vi "LJstreamM parse formula.vi"(7 "Num Args":u32, 8 "error in (no error)":errorcluster, 11 "Input Formula":string) -> (0 "error out":errorcluster, 2 "Output Formula Arguments":string[](array[string]), 3 "Output Formula":string)   [LabVIEW 2022 SP3]
doc: "Similar to the Formula Node function, but with variables that can be entered on the front panel."
panel:
  out "before substring 2":string
  out "before substring":string
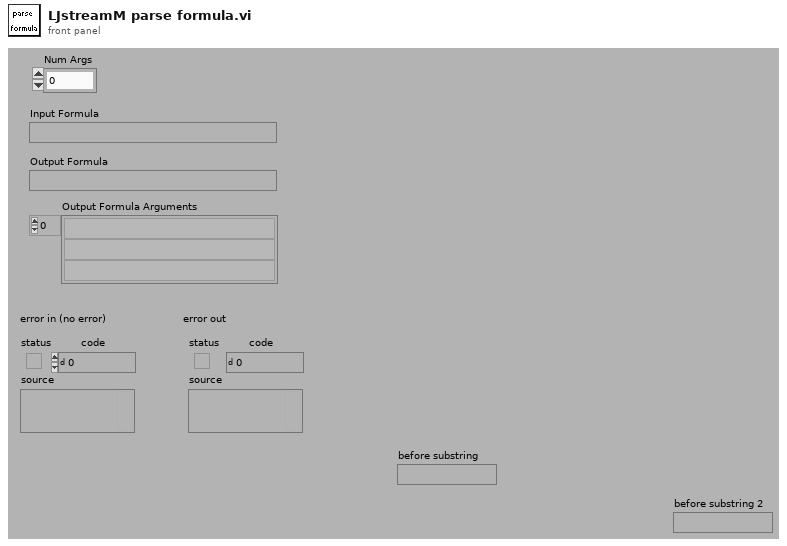
[diagram p1: front panel]
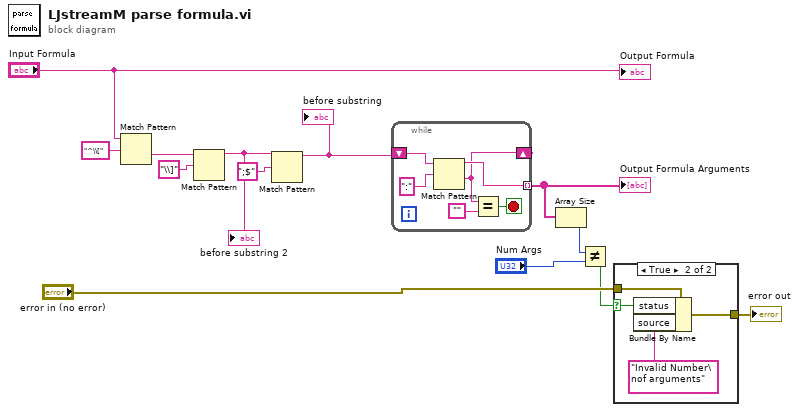
[diagram p0: block diagram]
diagram:
  n1 = Match Pattern(string="Input Formula", regular expression="^\\[") -> (after substring=w11:string)  [unwired: 1 in, 3 out]
  n2 = Match Pattern(string=w11, regular expression="\\]") -> (before substring=w2:string)  [unwired: 1 in, 3 out]
  "before substring 2" <- w2
  n3 = Match Pattern(string=w2, regular expression=";$") -> (before substring=w1:string)  [unwired: 1 in, 3 out]
  "before substring" <- w1
  n4 = while {
    shift-right: [w15] -> _
    shift-left: w1 -> [w19]
    tunnel: [w17] -> w9 mode=indexing
    stop <- w14 stop-if-true
    n5 = Match Pattern(string=w19, regular expression=":" ("search string/char (-)")) -> (before substring=w17:string, after substring=w15:string)  [unwired: 1 in, 2 out]
    n6 = Equal?(x=w15, y="") -> (x = y?=w14:bool)
  }
  "Output Formula Arguments" <- w9
  n7 = Array Size(array=w9) -> (size(s)=w8:i32)
  n8 = Not Equal?(x=w8, y="Num Args") -> (x != y?=w5:bool)
  n9 = case shown="True" w5 {
    selector: w5 -> [_ w22]
    tunnel: "error in (no error)" -> [w20 w24]
    tunnel: [w20 w21] -> w4
    frame False {
    }
    frame True {
      n10 = Bundle By Name(cluster=w24, "status"=w22, "source"="Invalid Number\nof arguments") -> (w21:errorcluster)
    }
  }
  "error out" <- w4
  "Output Formula" <- "Input Formula"
